vi "EOL CAN_Enable_Parametric_Mode.vi"(8 "Error in":errorcluster, 10 "Read Session in":refnum<k21>, 11 "Write Session in":refnum<k21>) -> (0 "Error out":errorcluster, 2 "debug log":string[][](array[string]), 3 "Response Good?":bool)   [LabVIEW 2014]
uses:
  <vilib>/xnet/xnet.llb/XNET Frame CAN.ctl
  <vilib>/xnet/xnet.llb/XNET Frame Type CAN.ctl
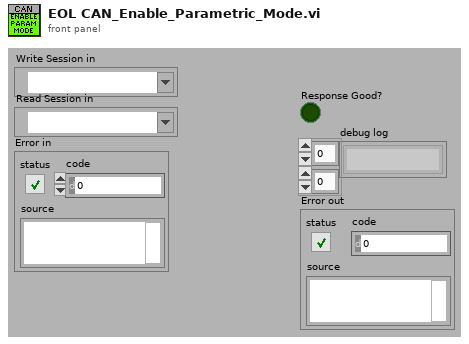
[diagram p1: front panel]
types:
  T1 = typedef "XNET Frame CAN.ctl" = cluster{"timestamp":timestamp, "payload":u8[], "identifier":u32, "type":T2, "extended?":bool, "echo?":bool}
  T2 = typedef "XNET Frame Type CAN.ctl" = u8
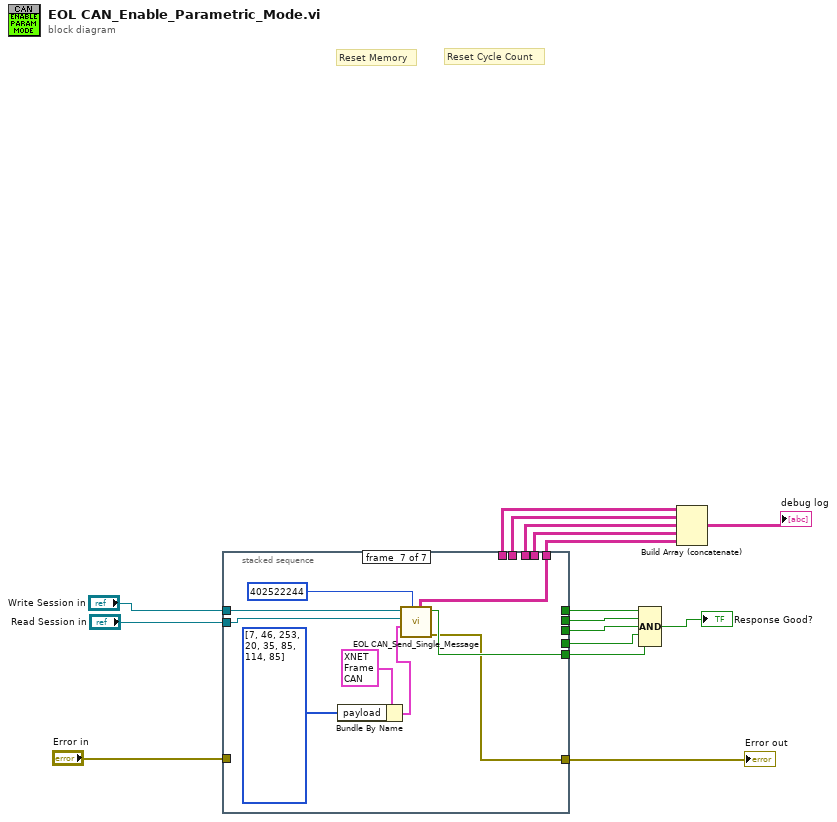
[diagram p0: block diagram]
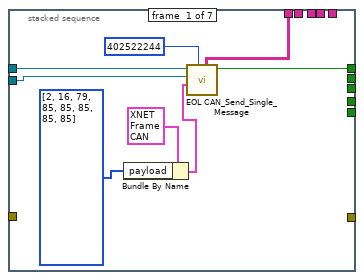
[diagram p2: hidden frame]
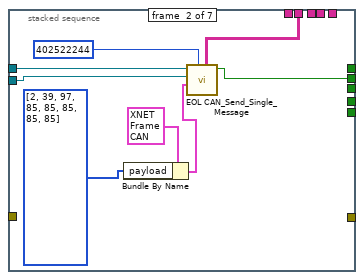
[diagram p3: hidden frame]
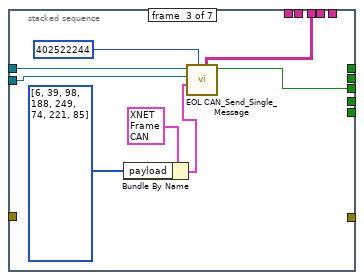
[diagram p4: hidden frame]
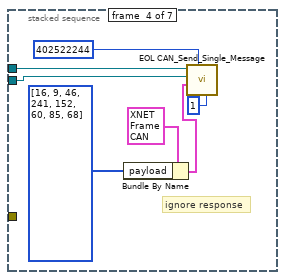
[diagram p5: hidden frame]
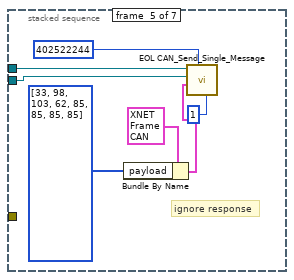
[diagram p6: hidden frame]
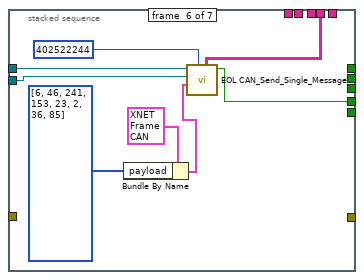
[diagram p7: hidden frame]
diagram:
  # "Reset Memory"
  # "Reset Cycle Count"
  n1 = stacked-sequence {
    tunnel: [w24 _ _ _ _ _ _] -> w16
    tunnel: [w23 _ _ _ _ _ _] -> w14
    tunnel: "Write Session in" -> [w22 w32 w40 w47 w54 w62 w71]
    tunnel: "Read Session in" -> [w21 w31 w39 w46 w53 w61 w70]
    tunnel: [_ w26 _ _ _ _ _] -> w10
    tunnel: [_ w25 _ _ _ _ _] -> w9
    tunnel: [_ _ w34 _ _ _ _] -> w8
    tunnel: [_ _ w33 _ _ _ _] -> w7
    tunnel: [_ _ _ _ _ w56 _] -> w6
    tunnel: [_ _ _ _ _ w55 _] -> w5
    tunnel: [_ _ _ _ _ _ w65] -> w4
    tunnel: [_ _ _ _ _ _ w64] -> w3
    tunnel: "Error in" -> [_ _ _ _ _ _ _]
    tunnel: [_ _ _ _ _ _ w63] -> w1
    frame #0 {
      n2 = Bundle By Name(cluster=T1 {"timestamp"=timestamp(0 s since 1904-01-01), "payload"=[2, 39, 3, 85, 85, 85, 85, 85], "identifier"=402391172, "type"=8, "extended?"=TRUE, "echo?"=FALSE} ("Tx CAN frame"), "payload"=u8[] [2, 16, 79, 85, 85, 85, 85, 85] ("Transmit Data 2")) -> (w19:T1)
      n3 = call "EOL CAN_Send_Single_Message.vi"("Rx Arbitration Id"=u32 402522244, "Tx CAN frame"=w19, "Read Session in"=w21, "Write Session in"=w22) -> ("Response Good?"=w24:bool, "TxRx Data"=w23:string[][])  [unwired: 3 in, 3 out]
    }
    frame #1 {
      n4 = Bundle By Name(cluster=T1 {"timestamp"=timestamp(0 s since 1904-01-01), "payload"=[2, 39, 3, 85, 85, 85, 85, 85], "identifier"=402391172, "type"=8, "extended?"=TRUE, "echo?"=FALSE} ("Tx CAN frame"), "payload"=u8[] [2, 39, 97, 85, 85, 85, 85, 85] ("Transmit Data 2")) -> (w30:T1)
      n5 = call "EOL CAN_Send_Single_Message.vi"("Rx Arbitration Id"=u32 402522244, "Tx CAN frame"=w30, "Read Session in"=w31, "Write Session in"=w32) -> ("Response Good?"=w25:bool, "TxRx Data"=w26:string[][])  [unwired: 3 in, 3 out]
    }
    frame #2 {
      n6 = Bundle By Name(cluster=T1 {"timestamp"=timestamp(0 s since 1904-01-01), "payload"=[2, 39, 3, 85, 85, 85, 85, 85], "identifier"=402391172, "type"=8, "extended?"=TRUE, "echo?"=FALSE} ("Tx CAN frame"), "payload"=u8[] [6, 39, 98, 188, 249, 74, 221, 85] ("Transmit Data 2")) -> (w38:T1)
      n7 = call "EOL CAN_Send_Single_Message.vi"("Rx Arbitration Id"=u32 402522244, "Tx CAN frame"=w38, "Read Session in"=w39, "Write Session in"=w40) -> ("Response Good?"=w33:bool, "TxRx Data"=w34:string[][])  [unwired: 3 in, 3 out]
    }
    frame #3 {
      # "ignore response"
      n8 = Bundle By Name(cluster=T1 {"timestamp"=timestamp(0 s since 1904-01-01), "payload"=[2, 39, 3, 85, 85, 85, 85, 85], "identifier"=402391172, "type"=8, "extended?"=TRUE, "echo?"=FALSE} ("Tx CAN frame"), "payload"=u8[] [16, 9, 46, 241, 152, 60, 85, 68] ("Transmit Data 2")) -> (w45:T1)
      n9 = call "EOL CAN_Send_Single_Message.vi"("Retries"=1, "Rx Arbitration Id"=u32 402522244, "Tx CAN frame"=w45, "Read Session in"=w46, "Write Session in"=w47) -> ()  [unwired: 2 in, 5 out]
    }
    frame #4 {
      # "ignore response"
      n10 = Bundle By Name(cluster=T1 {"timestamp"=timestamp(0 s since 1904-01-01), "payload"=[2, 39, 3, 85, 85, 85, 85, 85], "identifier"=402391172, "type"=8, "extended?"=TRUE, "echo?"=FALSE} ("Tx CAN frame"), "payload"=u8[] [33, 98, 103, 62, 85, 85, 85, 85] ("Transmit Data 2")) -> (w52:T1)
      n11 = call "EOL CAN_Send_Single_Message.vi"("Retries"=1, "Rx Arbitration Id"=u32 402522244, "Tx CAN frame"=w52, "Read Session in"=w53, "Write Session in"=w54) -> ()  [unwired: 2 in, 5 out]
    }
    frame #5 {
      n12 = Bundle By Name(cluster=T1 {"timestamp"=timestamp(0 s since 1904-01-01), "payload"=[2, 39, 3, 85, 85, 85, 85, 85], "identifier"=402391172, "type"=8, "extended?"=TRUE, "echo?"=FALSE} ("Tx CAN frame"), "payload"=u8[] [6, 46, 241, 153, 23, 2, 36, 85] ("Transmit Data 2")) -> (w60:T1)
      n13 = call "EOL CAN_Send_Single_Message.vi"("Rx Arbitration Id"=u32 402522244, "Tx CAN frame"=w60, "Read Session in"=w61, "Write Session in"=w62) -> ("Response Good?"=w55:bool, "TxRx Data"=w56:string[][])  [unwired: 3 in, 3 out]
    }
    frame #6 {
      n14 = Bundle By Name(cluster=T1 {"timestamp"=timestamp(0 s since 1904-01-01), "payload"=[2, 39, 3, 85, 85, 85, 85, 85], "identifier"=402391172, "type"=8, "extended?"=TRUE, "echo?"=FALSE} ("Tx CAN frame"), "payload"=u8[] [7, 46, 253, 20, 35, 85, 114, 85] ("Transmit Data 2")) -> (w69:T1)
      n15 = call "EOL CAN_Send_Single_Message.vi"("Rx Arbitration Id"=u32 402522244, "Tx CAN frame"=w69, "Read Session in"=w70, "Write Session in"=w71) -> ("Error out"=w63:errorcluster, "Response Good?"=w64:bool, "TxRx Data"=w65:string[][])  [unwired: 3 in, 2 out]
    }
  }
  "Error out" <- w1
  n16 = Compound Arithmetic op=AND(w16, w9, w7, w5, w3) -> (→"Response Good?":bool)
  n17 = Build Array (concatenate)(w14, w10, w8, w6, w4) -> (→"debug log":string[][])
